vi "Limit Switch Config.vi"(11 "DIO Channel":T1) -> ()   [LabVIEW 2012]
uses:
  <vilib>/Rock Robotics/SystemInterfaces/DIO/FPGA_DIOChannel.ctl
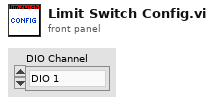
[diagram p1: front panel]
types:
  T1 = typedef "FPGA_DIOChannel.ctl" = enum8{"DIO 1", "DIO 2", "DIO 3", "DIO 4", "DIO 5", "DIO 6", "DIO 7", "DIO 8", "DIO 9", "DIO 10", "DIO 11", "DIO 12", "DIO 13", "DIO 14", "Invalid"}
  T2 = typedef "WPI_DigitalInputDevRef.ctl" = cluster{"DevStatus":errorcluster, "DIO Channel":T1, "Digital Module":T3}
  T3 = typedef "FPGA_TypedefDigitalModule.ctl" = enum16{"Digital Module 1", "Digital Module 2"}
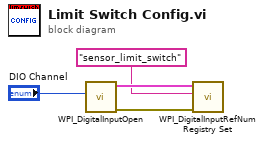
[diagram p0: block diagram]
diagram:
  n1 = call <vilib>:"WPI_DigitalInputOpen.vi"("DIO Channel"="DIO Channel") -> ("error out"=w3:errorcluster, "DigitalInputDevRef"=w4:T2)  [unwired: 9 in]
  n2 = call <vilib>:"WPI_DigitalInputRefNum Registry Set.vi"("error in (no error)"=w3, "refnum name"="sensor_limit_switch", "DigitalInputDevRef"=w4) -> ()  [unwired: 7 in, 2 out]
